vi "PPM Modulator.vi"(0 "Input level":dbl(slide)=50.0 scale=50.0..310.0, 5 "Carrier Frequency(Hz)":dbl(slide)=1000.0 scale=20.0..8000000000.0, 11 "error in (no error)":errorcluster) -> (4 "PPM with Sync":waveform(dbl)(graph), 6 "Sampling Info":cluster{"Fs":dbl, "#s":dbl}, 15 "error out":errorcluster)   [LabVIEW 2013]
uses:
  <vilib>/measure/NI_MABase.lvlib
panel:
  # "PULSE POSITION MODULATION"
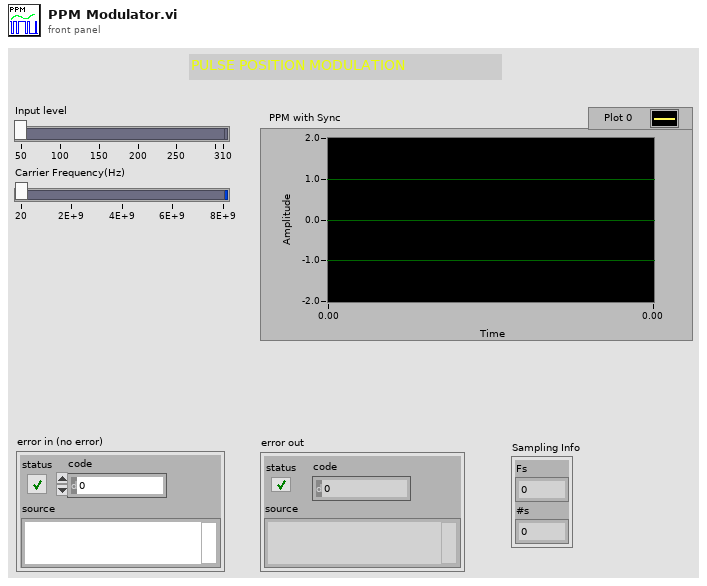
[diagram p1: front panel]
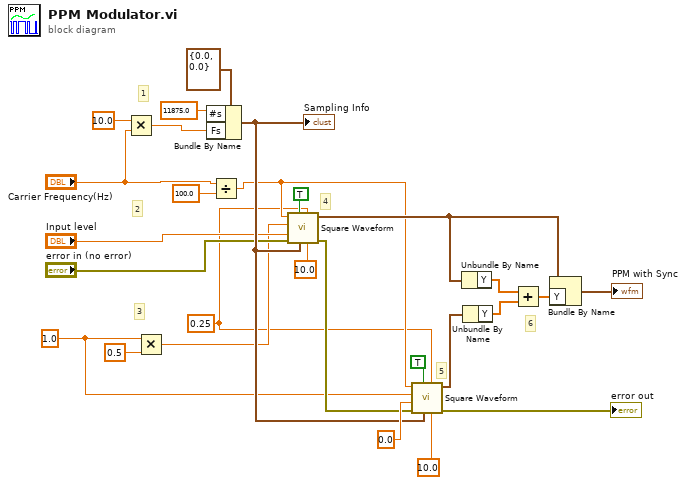
[diagram p0: block diagram]
diagram:
  w1 = 0.25
  w3 = 1.0 ("amplitude")
  # "6"
  # "5"
  # "4"
  # "3"
  # "1"
  # "2"
  n1 = Multiply(x=10.0, y="Carrier Frequency(Hz)") -> (x*y=w6:dbl)
  n2 = Multiply(x=w3, y=0.5) -> (x*y=w4:dbl)
  n3 = Bundle By Name(cluster=cluster{"Fs":dbl, "#s":dbl} {"Fs"=0.0, "#s"=0.0}, "#s"=11875.0, "Fs"=w6) -> (w15:cluster{"Fs":dbl, "#s":dbl})
  "Sampling Info" <- w15
  n4 = Divide(x="Carrier Frequency(Hz)", y=100.0) -> (x/y=w5:dbl)
  n5 = call <vilib>:"Square Waveform.vi"("duty cycle (%)"=10.0, "offset"=w1, "sampling info"=w15, "reset signal"=TRUE, "error in (no error)"="error in (no error)", "phase"="Input level", "amplitude"=w4, "frequency"=w5) -> ("error out"=w14:errorcluster, "signal out"=w18:waveform(dbl))  [unwired: 2 in]
  n6 = call <vilib>:"Square Waveform.vi"("duty cycle (%)"=10.0, "offset"=w1, "sampling info"=w15, "reset signal"=TRUE, "error in (no error)"=w14, "phase"=0.0, "amplitude"=w3, "frequency"=w5) -> ("error out"=→"error out":errorcluster, "signal out"=w19:waveform(dbl))  [unwired: 2 in]
  n7 = Unbundle By Name(w18) -> ("Y"=w22:dbl[])
  n8 = Unbundle By Name(w19) -> ("Y"=w21:dbl[])
  n9 = Add(x=w22, y=w21) -> (x+y=w20:dbl[])
  n10 = Bundle By Name(cluster=w18, "Y"=w20) -> (→"PPM with Sync":waveform(dbl))
